vi "Find Part Numbers.vi"() -> (3 "Part Numbers":string[](array[string]))   [LabVIEW 2018]
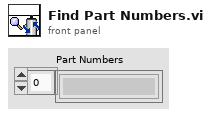
[diagram p1: front panel]
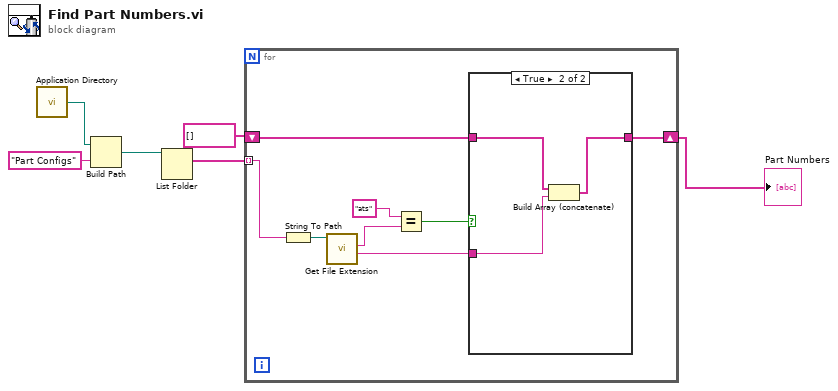
[diagram p0: block diagram]
diagram:
  n1 = call <vilib>:"Application Directory.vi"() -> ("Application Directory"=w5:path)
  n2 = Build Path(base path=w5, name or relative path="Part Configs") -> (appended path=w6:path)
  n3 = List Folder(path=w6) -> (filenames=w3:string[])  [unwired: 3 in, 3 out]
  n4 = for {
    tunnel: w3 -> [w12] mode=indexing
    shift-right: [w13] -> w1
    shift-left: string[] [] -> [w14]
    n5 = String To Path(string=w12) -> (path=w11:path)
    n6 = call <vilib>:"Get File Extension.vi"("file"=w11) -> ("filename without extension"=w10:string, "lowercase file extension"=w9:string)  [unwired: 6 in, 3 out]
    n7 = Equal?(x="ats", y=w9) -> (x = y?=w7:bool)
    n8 = case shown="True" w7 {
      tunnel: w14 -> [w15 w18]
      tunnel: [w15 w17] -> w13
      tunnel: w10 -> [_ w16]
      frame False {
      }
      frame True {
        n9 = Build Array (concatenate)(w18, w16) -> (w17:string[])
      }
    }
  }
  "Part Numbers" <- w1
